vi "ADAM6018_2.1.vi"(0 "ADAM6018_Command":enum16{"Open_Adam", "Read_Adam", "Close_Adam"}(ring)=enum."Close_Adam", 5 "ID_in":refnum<k5>, 7 "IP Address":string="192.168.0.165", 9 "Port":u16=502, 11 "error in (no error)":errorcluster) -> (4 "Temps":sgl[](array[numeric])=[22.212069, 20.758484], 6 "ADAM_ID":refnum<k5>, 15 "error out":errorcluster)   [LabVIEW 2012]
uses:
  nimodbus121/86/vi.lib/NI Modbus.llb/MB Modbus Command.ctl
panel:
  out "Slave Input Registers 2":u16[](array[numeric])=[1201, 1109, 16146] caption="Slave Input Registers (Read Only)"
  in  "Modbus Command":T1={"Function Code"=4, "Starting Address"=0, "Quantity"=3, "Data"=[], "Discrete"=[]} {"Function Code" items=["Read Coils"=1, "Read Discrete Inputs"=2, "Read Holding Registers"=3, "Read Input Registers"=4, "Write Single Coil"=5, "Write Single Register"=6, "Read Exception Status"=7, "Write Multiple Coils"=15, "Write Multiple Registers"=16]}
  # "ADAM 6018"
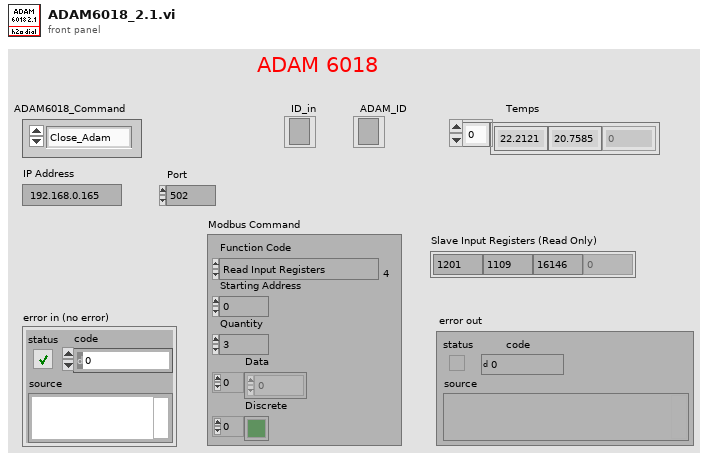
[diagram p1: front panel]
types:
  T1 = typedef "MB Modbus Command.ctl" = cluster{"Function Code":u8, "Starting Address":u16, "Quantity":u16, "Data":u16[], "Discrete":bool[]}
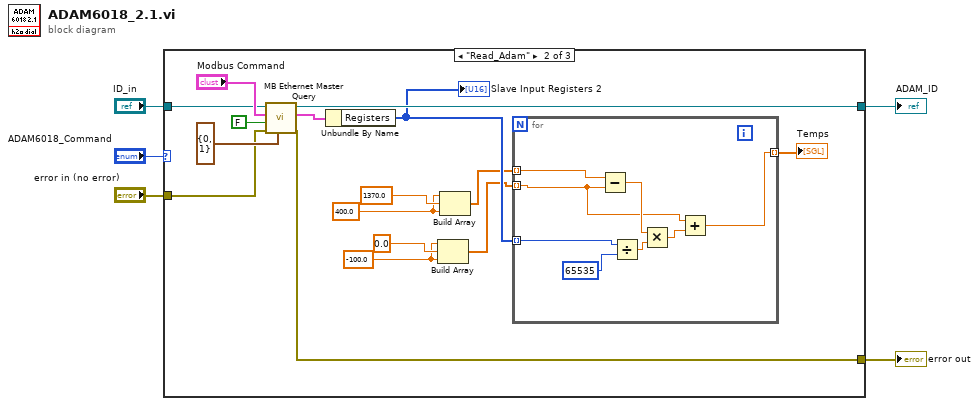
[diagram p0: block diagram]
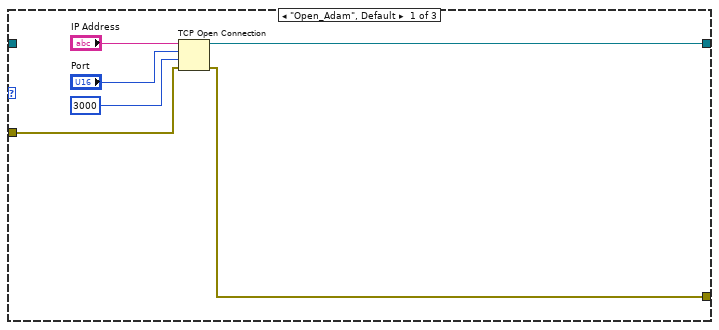
[diagram p2: hidden frame]
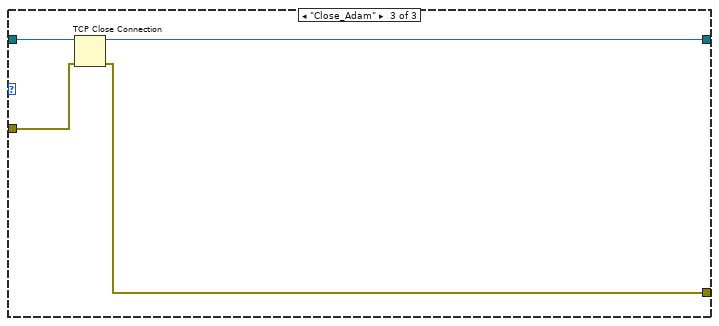
[diagram p3: hidden frame]
diagram:
  n1 = case shown="\"Read_Adam\"" "ADAM6018_Command" {
    tunnel: [w8 w23 w38] -> w4
    tunnel: "ID_in" -> [_ w19 w39]
    tunnel: [w7 w20 w36] -> w3
    tunnel: "error in (no error)" -> [w6 w22 w37]
    frame "Open_Adam", Default {
      n2 = TCP Open Connection(address="IP Address", remote port or service name="Port", timeout ms (60000)=3000, error in (no error)=w6) -> (connection ID=w8:refnum<k5>, error out=w7:errorcluster)  [unwired: 1 in]
    }
    frame "Read_Adam" {
      w12 = 400.0 ("element")
      w13 = -100.0 ("element")
      n3 = call "MB Ethernet Master Query.vi"("MBAP Header"=cluster{"Transaction ID":u16, "Unit ID":u8} {"Transaction ID"=0, "Unit ID"=1}, "error in (no error)"=w22, "Use MODBUS Data Unit?"=FALSE, "Modbus Command"="Modbus Command", "TCP Connection Refnum in"=w19) -> ("error out"=w20:errorcluster, "Registers"=w26:cluster{"Registers":u16[], "Discrete":bool[]}, "TCP Connection Refnum (dup)"=w23:refnum<k5>)  [unwired: 2 in, 2 out]
      n4 = Unbundle By Name(w26) -> ("Registers"=w16:u16[])
      "Slave Input Registers 2" <- w16
      n5 = Build Array(w13, 0.0 ("element"), w13) -> (w15:dbl[])
      n6 = Build Array(w12, 1370.0 ("element"), w12) -> (w14:dbl[])
      n7 = for {
        tunnel: [w28] -> w21 mode=indexing
        tunnel: w16 -> [w31] mode=indexing
        tunnel: w15 -> [w30] mode=indexing
        tunnel: w14 -> [w29] mode=indexing
        n8 = Subtract(x=w29, y=w30) -> (x-y=w34:dbl)
        n9 = Divide(x=w31, y=u16 65535) -> (x/y=w33:dbl)
        n10 = Multiply(x=w34, y=w33) -> (x*y=w35:dbl)
        n11 = Add(x=w30, y=w35) -> (x+y=w28:dbl)
      }
      "Temps" <- w21
    }
    frame "Close_Adam" {
      n12 = TCP Close Connection(connection ID=w39, error in (no error)=w37) -> (connection ID out=w38:refnum<k5>, error out=w36:errorcluster)  [unwired: 1 in]
    }
  }
  "error out" <- w3
  "ADAM_ID" <- w4
